vi "Add Parameter.vi"(8 "error in":errorcluster, 10 "parameter":T2={"name"="", "direction"=enum."Rx", "default value"=0.0, "unit"="", "Parameter"={"start index"=0, "size"=8, "encoding"=enum."BCD", "signed"=FALSE, "scale multiplier"=1.0, "scale offset"=0.0}}, 11 "word ref":T1 format="%.0x") -> (0 "error out":errorcluster, 2 "parameter ref":T1 format="%.0x", 3 "word ref out":T1 format="%.0x")   [LabVIEW 2020, in "Ballard ARINC 429 Scripting.lvlib"]
uses:
  Ballard ARINC 429 Scripting.lvlib
  Constants.vi
  <vilib>/NI VeriStand/Custom Device API/Custom Device API.lvlib
  <vilib>/NI VeriStand/Custom Device API/Custom Device Channel Type.ctl
  <vilib>/NI VeriStand/Custom Device API/Custom Device Channel.ctl
  <vilib>/NI VeriStand/Custom Device API/Custom Device Item Ref.ctl
  Encoding and Decoding/Encoding.ctl
  Encoding and Decoding/Encoding and Decoding.lvlib
  Shared/Parameter Definition.ctl
  Shared/Direction.ctl
  Shared/VS Channel Definition for Parameter.ctl
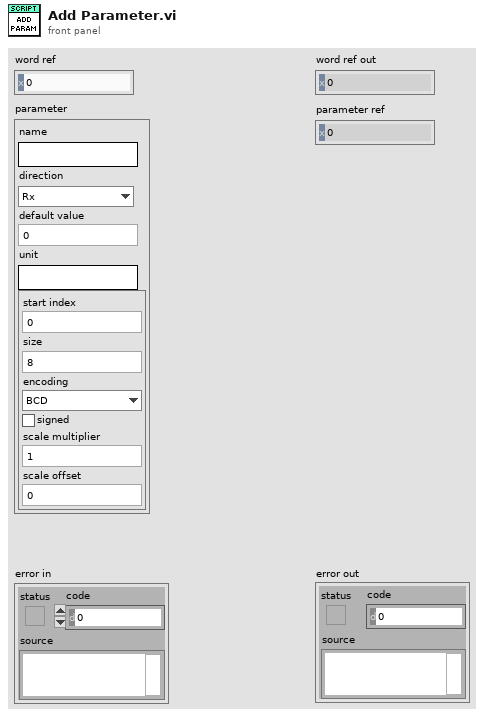
[diagram p1: front panel]
types:
  T1 = typedef "Custom Device API.lvlib/Custom Device Item Ref.ctl" = u64
  T2 = typedef "VS Channel Definition for Parameter.ctl" = cluster{"name":string, "direction":T3, "default value":dbl, "unit":string, "Parameter":T4}
  T3 = typedef "Direction.ctl" = enum16{"Rx", "Tx"}
  T4 = typedef "Parameter Definition.ctl" = cluster{"start index":i32, "size":i32, "encoding":T5, "signed":bool, "scale multiplier":dbl, "scale offset":dbl}
  T5 = typedef "Encoding and Decoding.lvlib/Encoding.ctl" = enum16{"BNR", "BCD", "Discrete"}
  T6 = typedef "Custom Device API.lvlib/Custom Device Channel.ctl" = cluster{"Type":T7, "Units":string, "Default Value":dbl, "Faultable":bool, "Scalable":bool}
  T7 = typedef "Custom Device API.lvlib/Custom Device Channel Type.ctl" = enum16{"Input", "Output"}
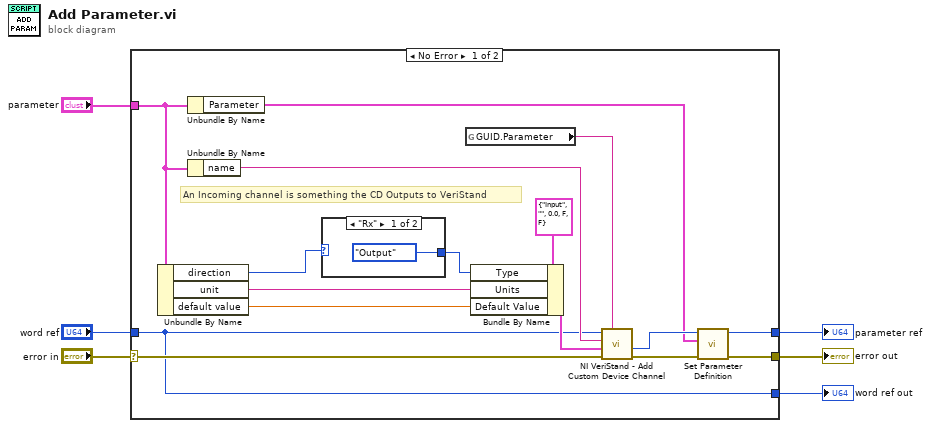
[diagram p0: block diagram]
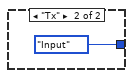
[diagram p2: hidden frame]
diagram:
  n1 = case shown="No Error" "error in" {
    selector: "error in" -> [w22 w26]
    tunnel: [w10 w26] -> w5
    tunnel: "word ref" -> [w14 w25]
    tunnel: [w11 _] -> w3
    tunnel: "parameter" -> [w16 _]
    tunnel: [w14 w25] -> w1
    frame No Error {
      # "An Incoming channel is something the CD Outputs to VeriStand"
      n2 = Unbundle By Name(w16) -> ("direction"=w8:T3, "unit"=w17:string, "default value"=w15:dbl)
      n3 = Unbundle By Name(w16) -> ("Parameter"=w9:T4)
      n4 = Unbundle By Name(w16) -> ("name"=w20:string)
      n5 = case shown="\"Rx\"" w8 {
        tunnel: [Custom_Device_Channel_Type."Output" ("Type") Custom_Device_Channel_Type."Input" ("Type")] -> w7
        frame "Rx" {
        }
        frame "Tx" {
        }
      }
      n6 = global read "Constants.vi" "GUID.Parameter"() -> (w21:string)
      n7 = Bundle By Name(cluster=T6 {"Type"=enum."Input", "Units"="", "Default Value"=0.0, "Faultable"=FALSE, "Scalable"=FALSE} ("Channel"), "Type"=w7, "Units"=w17, "Default Value"=w15) -> (w18:T6)
      n8 = call <vilib>:"NI VeriStand - Add Custom Device Channel.vi"("GUID (Default Channel)"=w21, "error in (no error)"=w22, "Channel"=w18, "Channel Name"=w20, "Parent Ref in"=w14) -> ("error out"=w13:errorcluster, "Channel Ref"=w12:T1)  [unwired: 3 in, 2 out]
      n9 = call "Set Parameter Definition.vi"("error in"=w13, "parameter definition"=w9, "parameter ref in"=w12) -> ("error out"=w10:errorcluster, "parameter ref out"=w11:T1)  [unwired: 7 in]
    }
    frame Error {
    }
  }
  "parameter ref" <- w3
  "error out" <- w5
  "word ref out" <- w1
